vi "Setup AWG and Measure Capacitance Only_ER_Mod.vi"(4 "cleanup script":string="BeamsOff", 5 "setup script":string="PullDown41v", 6 "error in (no error)":errorcluster, 7 "VNAs Measurement Parameters":T1, 8 "Measurement Id":string="CMax", 9 "Semiconductor Module Context":T2) -> (0 "error out":errorcluster, 3 "Semiconductor Module Context Out":T2)   [LabVIEW 2013]
uses:
  <vilib>/NI_TestStand_SemiconductorModule/NI_TestStand_Semiconductor_Module.lvlibp/PinMap/General/SemiconductorModuleContext.ctl
  VNA/VNAs Measurement Parameters.ctl
  <instrlib>/niHSDIO/niHSDIO.llb/niHSDIO_ctl Trigger Script - trigID Values (Ring).ctl
  <vilib>/NI_TestStand_SemiconductorModule/NI_TestStand_Semiconductor_Module.lvlibp
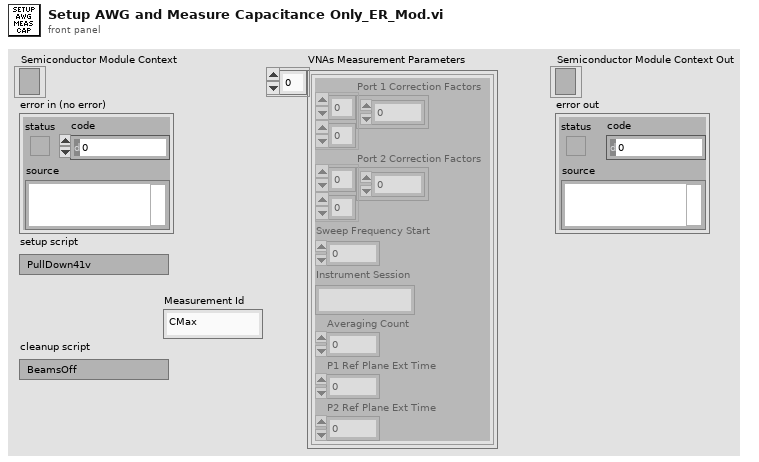
[diagram p1: front panel]
types:
  T1 = typedef "VNAs Measurement Parameters.ctl" = cluster{"Port 1 Correction Factors":cdb[][], "Port 2 Correction Factors":cdb[][], "Sweep Frequency Start":dbl, "Instrument Session":string, "Averaging Count":i32, "P1 Ref Plane Ext Time":dbl, "P2 Ref Plane Ext Time":dbl}[]
  T2 = typedef "NI_TestStand_Semiconductor_Module.lvlibp/SemiconductorModuleContext.ctl" = refnum<k7>
  T3 = typedef "niHSDIO_ctl Trigger Script - trigID Values (Ring).ctl" = string
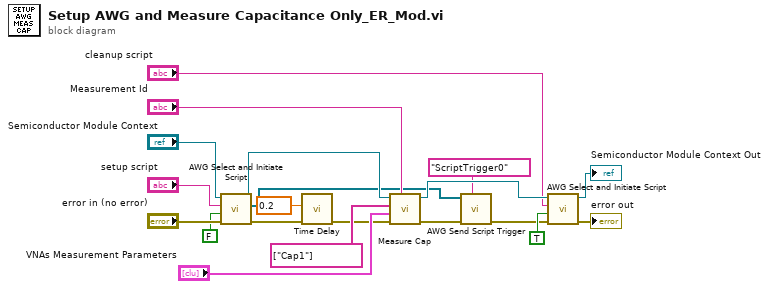
[diagram p0: block diagram]
diagram:
  n1 = call "AWG Select and Initiate Script.vi"("error in (no error)"="error in (no error)", "Wait for Completion"=FALSE, "script name"="setup script", "Semiconductor Module Context"="Semiconductor Module Context") -> ("error out"=w16:errorcluster, "Sessions Out"=w1:refnum<k15>[], "Semiconductor Module Context Out"=w12:T2)  [unwired: 5 in]
  n2 = call "Time Delay"("error in (no error)"=w16, "Delay Time (s)"=0.2) -> ("error out"=w6:errorcluster)  [unwired: 9 in]
  n3 = call "Measure Cap.vi"("Measurement Id"="Measurement Id", "error in (no error)"=w6, "VNAs Measurement Parameters"="VNAs Measurement Parameters", "Pins"=string[] ["Cap1"] ("Capacitance Pins"), "Semiconductor Module Context"=w12) -> ("error out"=w3:errorcluster, "Semiconductor Module Context Out"=w13:T2)  [unwired: 4 in, 1 out]
  n4 = call "AWG Send Script Trigger.vi"("trigger id (script trigger 0)"=T3 "ScriptTrigger0", "error in (no error)"=w3, "AWG Sessions In"=w1) -> ("error out"=w2:errorcluster)  [unwired: 7 in, 1 out]
  n5 = call "AWG Select and Initiate Script.vi"("error in (no error)"=w2, "Wait for Completion"=TRUE, "script name"="cleanup script", "Semiconductor Module Context"=w13) -> ("error out"=→"error out":errorcluster, "Semiconductor Module Context Out"=→"Semiconductor Module Context Out":T2)  [unwired: 5 in, 1 out]
